vi "ChangeFileExtension.vi"(10 "NewFileExtension":string, 11 "Path to was selected by user":path) -> (3 "appended path":path)   [LabVIEW 2013]
uses:
  <vilib>/regexp/Match Regular Expression.xnode
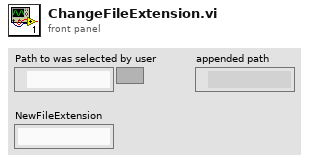
[diagram p1: front panel]
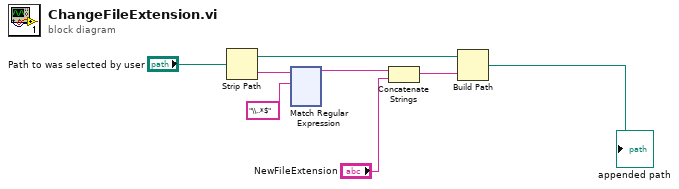
[diagram p0: block diagram]
diagram:
  n1 = Strip Path(path="Path to was selected by user") -> (stripped path=w6:path, name=w1:string)
  n2 = xnode "Match Regular Expression"("input string"=w1, "regular expression"="\\..*$") -> ("before match"=w4:string)  [unwired: 4 in, 4 out]
  n3 = Concatenate Strings(w4, "NewFileExtension") -> (w7:string)
  n4 = Build Path(base path=w6, name or relative path=w7) -> (appended path=→"appended path":path)
